vi "HelloWorld.vi"() -> ()   [LabVIEW 2018]
panel:
  in  "message":string="Hello World!"
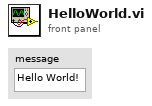
[diagram p1: front panel]
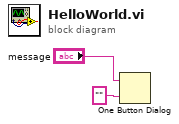
[diagram p0: block diagram]
diagram:
  n1 = One Button Dialog(message="message", button name ("OK")="") -> ()  [unwired: 1 out]
